vi "CheckDelays.vi"(9 "current level":i32, 10 "rule":T3, 11 "cache in":T1) -> (1 "update":bool, 3 "cache out":T1)   [LabVIEW 2017, in "TrendAlarm.lvlib"]
uses:
  <vilib>/addons/InsightCM/Devices/Shared/Common/TrendAlarm/TrendAlarm.lvlib
  <vilib>/addons/InsightCM/MessageBus/Base/controls/TrendAlarmRule.ctl
  <vilib>/addons/InsightCM/MessageBus/Base/controls/TrendAlarmLevel.ctl
  <vilib>/addons/InsightCM/MessageBus/Base/controls/AlarmAction.ctl
  <vilib>/addons/InsightCM/MessageBus/Base/controls/KeyValuePair.ctl
  <vilib>/addons/InsightCM/Devices/Shared/Common/TrendAlarm/controls/TransitionCache.ctl
  <vilib>/addons/InsightCM/MessageBus/Base/controls/TrendAlarmTransition.ctl
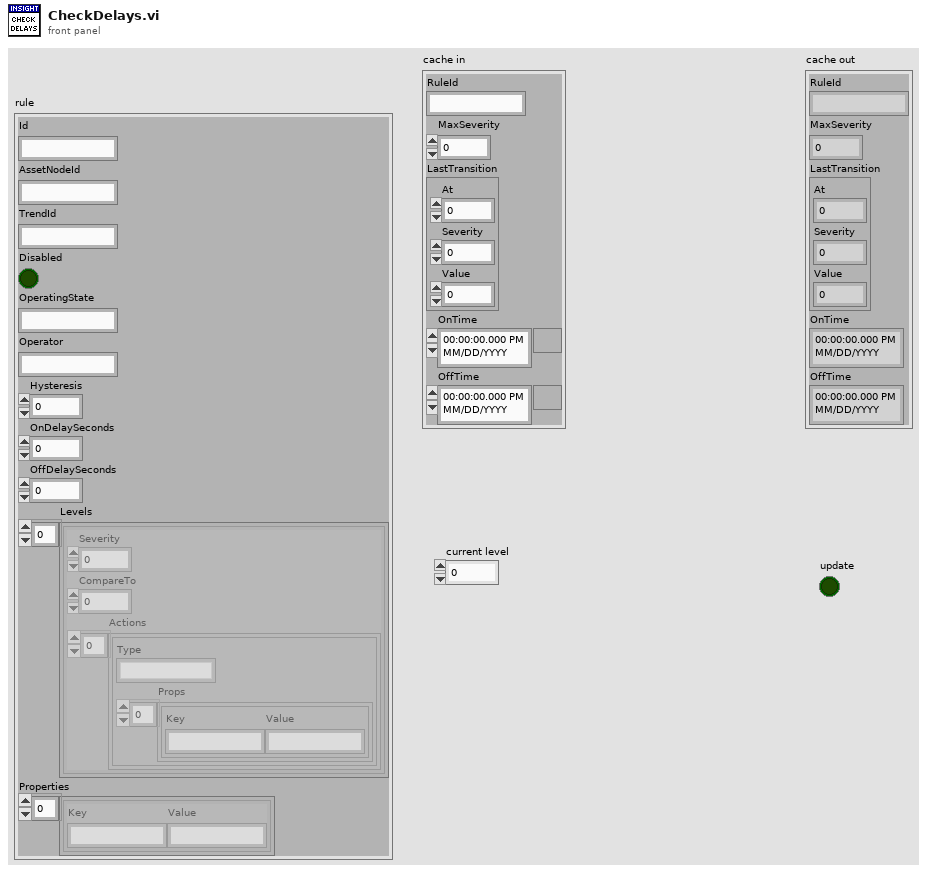
[diagram p1: front panel]
types:
  T1 = typedef "TrendAlarm.lvlib/TransitionCache.ctl" = cluster{"RuleId":string, "MaxSeverity":i32, "LastTransition":T2, "OnTime":timestamp, "OffTime":timestamp}
  T2 = typedef "TrendAlarmTransition.ctl" = cluster{"At":i64, "Severity":i32, "Value":dbl}
  T3 = typedef "TrendAlarmRule.ctl" = cluster{"Id":string, "AssetNodeId":string, "TrendId":string, "Disabled":bool, "OperatingState":string, "Operator":string, "Hysteresis":dbl, "OnDelaySeconds":dbl, "OffDelaySeconds":dbl, "Levels":T4[], "Properties":T6[]}
  T4 = typedef "TrendAlarmLevel.ctl" = cluster{"Severity":i32, "CompareTo":dbl, "Actions":T5[]}
  T5 = typedef "AlarmAction.ctl" = cluster{"Type":string, "Props":T6[]}
  T6 = typedef "KeyValuePair.ctl" = cluster{"Key":string, "Value":string}
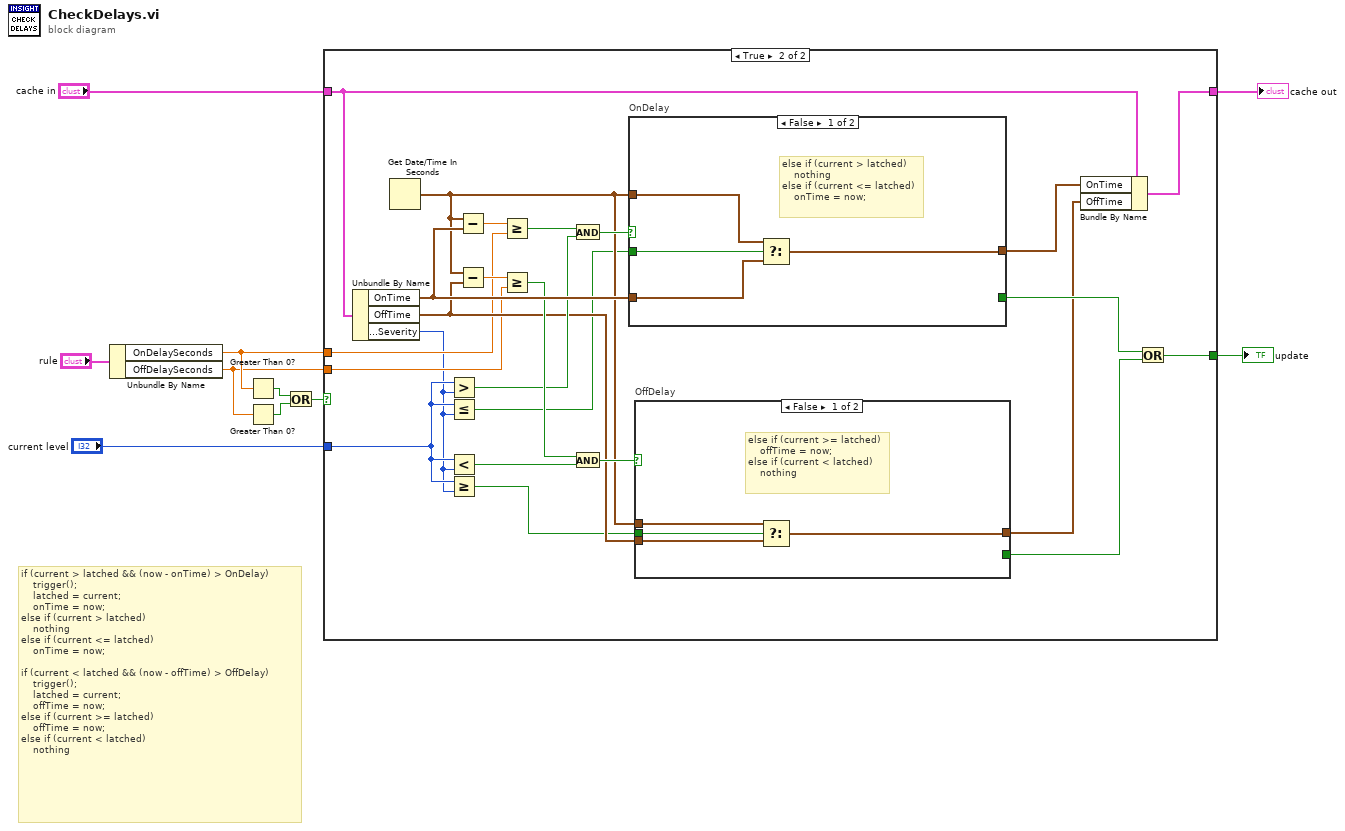
[diagram p0: block diagram]
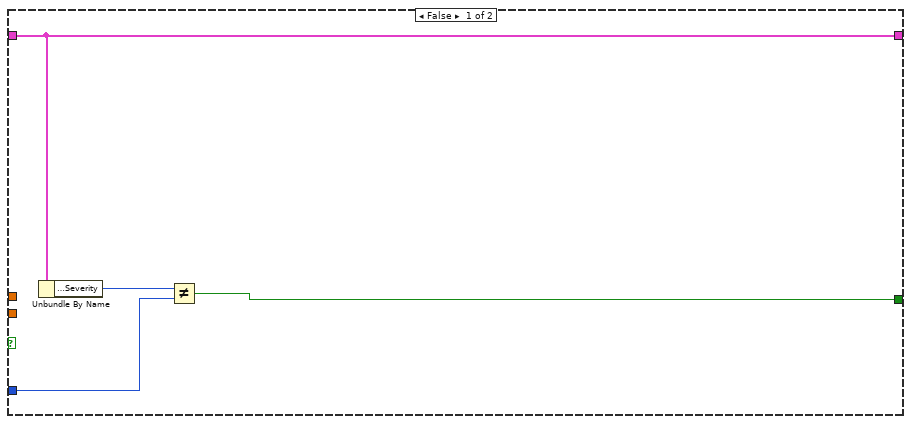
[diagram p2: hidden frame]
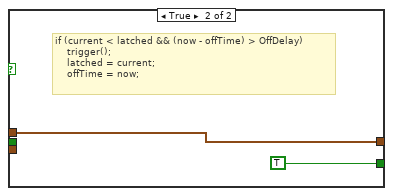
[diagram p3: hidden frame]
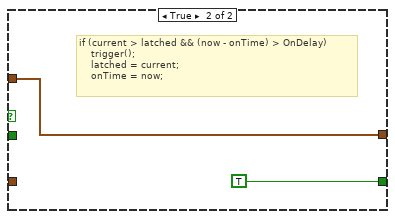
[diagram p4: hidden frame]
diagram:
  # "if (current > latched && (now - onTime) > OnDelay)\n   \ttrigger();\n  \t latched = current;\n \t \tonTime = now;\nelse if (current > latched)\n \t \tnothing\nelse if (current <= latched)\n \t \tonTime = now;\n\nif (current < latched && (now - offTime) > OffDelay)\n \t \ttrigger();\n \t \tlatched = current;\n \t \toffTime = now;\nelse if (current >= latched)\n \t \toffTime = now;\nelse if (current < latched)\n \t \tnothing"
  n1 = Unbundle By Name("rule") -> ("OnDelaySeconds"=w3:dbl, "OffDelaySeconds"=w2:dbl)
  n2 = Greater Than 0?(x=w3) -> (x > 0?=w5:bool)
  n3 = Greater Than 0?(x=w2) -> (x > 0?=w4:bool)
  n4 = Or(x=w5, y=w4) -> (x .or. y?=w1:bool)
  n5 = case shown="True" w1 {
    tunnel: "current level" -> [w12 w17]
    tunnel: [w11 w25] -> w8
    tunnel: "cache in" -> [w14 w24]
    tunnel: [w14 w21] -> w6
    tunnel: w3 -> [_ w20]
    tunnel: w2 -> [_ w19]
    frame False {
      n6 = Unbundle By Name(w14) -> ("LastTransition.Severity"=w13:i32)
      n7 = Not Equal?(x=w13, y=w12) -> (x != y?=w11:bool)
    }
    frame True {
      n8 = Unbundle By Name(w24) -> ("OnTime"=w34:timestamp, "OffTime"=w28:timestamp, "LastTransition.Severity"=w16:i32)
      n9 = Get Date/Time In Seconds() -> (seconds since 1Jan1904=w29:timestamp)
      n10 = Greater?(x=w17, y=w16) -> (0:w30:bool)
      n11 = Less Or Equal?(x=w17, y=w16) -> (x <= y?=w15:bool)
      n12 = Less?(x=w17, y=w16) -> (x < y?=w33:bool)
      n13 = Greater Or Equal?(x=w17, y=w16) -> (x >= y?=w18:bool)
      n14 = Subtract(x=w29, y=w34) -> (x-y=w38:dbl)
      n15 = Subtract(x=w29, y=w28) -> (x-y=w37:dbl)
      n16 = Greater Or Equal?(x=w38, y=w20) -> (x >= y?=w36:bool)
      n17 = Greater Or Equal?(x=w37, y=w19) -> (x >= y?=w31:bool)
      n18 = And(x=w36, y=w30) -> (x .and. y?=w35:bool)
      n19 = And(x=w31, y=w33) -> (x .and. y?=w32:bool)
      n20 = case "OnDelay" shown="False" w35 {
        tunnel: [_ TRUE] -> w27
        tunnel: [w45 w49] -> w23
        tunnel: w29 -> [w47 w49]
        tunnel: w15 -> [w48 _]
        tunnel: w34 -> [w46 _]
        frame False {
          # "else if (current > latched)\n \t \tnothing\nelse if (current <= latched)\n \t \tonTime = now;"
          n21 = Select(t=w47, s=w48, f=w46) -> (s? t:f=w45:timestamp)
        }
        frame True {
          # "if (current > latched && (now - onTime) > OnDelay)\n   \ttrigger();\n  \t latched = current;\n \t \tonTime = now;"
        }
      }
      n22 = case "OffDelay" shown="False" w32 {
        tunnel: [_ TRUE] -> w26
        tunnel: w18 -> [w42 _]
        tunnel: w29 -> [w41 w43]
        tunnel: w28 -> [w40 _]
        tunnel: [w39 w43] -> w22
        frame False {
          # "else if (current >= latched)\n \t \toffTime = now;\nelse if (current < latched)\n \t \tnothing"
          n23 = Select(t=w41, s=w42, f=w40) -> (s? t:f=w39:timestamp)
        }
        frame True {
          # "if (current < latched && (now - offTime) > OffDelay)\n \t \ttrigger();\n \t \tlatched = current;\n \t \toffTime = now;"
        }
      }
      n24 = Bundle By Name(cluster=w24, "OnTime"=w23, "OffTime"=w22) -> (w21:T1)
      n25 = Or(x=w27, y=w26) -> (x .or. y?=w25:bool)
    }
  }
  "cache out" <- w6
  "update" <- w8
